vi "CALC_FORM.vi"(0 "VISA IN":refnum<visa-resource-name>, 1 "Format":string(combo)="MLINear", 5 "error in":errorcluster, 7 "Channel":i32) -> (14 "VISA Out":refnum<visa-resource-name>, 19 "error out":errorcluster)   [LabVIEW 2018, in "PNA-X.lvlib"]
doc: "CALCulate<cnum>:FORMat <char> \n(Read-Write) Sets the display format for the measurement. \nSee Critical Note \nParameters \n<cnum> Channel number of the measurement. There must be a selected measurement \non that channel. If unspecified, <cnum> is set to 1. \n<char> Choose from: \nMLINear \nMLOGarithmic \nPHASe \nUPHase 'Unwrapped phase \nIMAGinary \nREAL \nPOLar \nSMITh \nSADMittance 'Smith Admittance \nSWR \nGDELay 'Group Delay \n1512\n\nExamples CALC:FORM MLIN \ncalculate2:format polar \nQuery Syntax CALCulate<cnum>:FORMat? \nReturn Type Character \nDefault MLINear \n1513\n\nCalculate:FSimulator Commands \nSpecifies settings and fixturing for Balanced Measurements. \nClick a blue keyword to view the command details. \nSee Also \nExample Programs \nSCPI Command Tree"
uses:
  PNA-X.lvlib
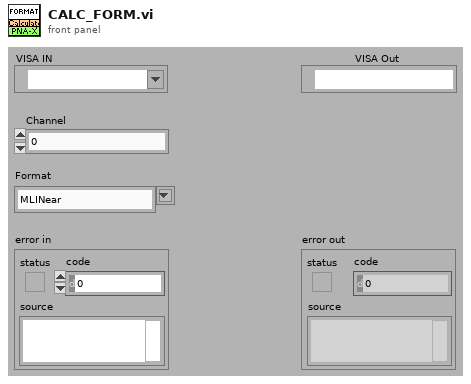
[diagram p1: front panel]
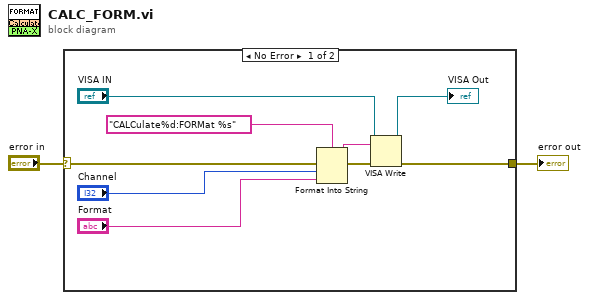
[diagram p0: block diagram]
diagram:
  n1 = case shown="No Error" "error in" {
    selector: "error in" -> [w11 w12]
    tunnel: [w6 w12] -> w1
    frame No Error {
      n2 = Format Into String(format string="CALCulate%d:FORMat %s" ("Cmdline"), error in=w11, "Channel", "Format") -> (resulting string=w9:string, error out=w10:errorcluster)  [unwired: 1 in]
      n3 = VISA Write(VISA resource name="VISA IN", write buffer=w9, error in (no error)=w10) -> (VISA resource name out=→"VISA Out":refnum<visa-resource-name>, error out=w6:errorcluster)  [unwired: 1 out]
    }
    frame Error {
    }
  }
  "error out" <- w1
